vi "Blocking Read After Fulfill.vi"(8 "error in (no error)":errorcluster) -> (0 "error out":errorcluster)   [LabVIEW 2017, in "Unit Tests.lvlib"]
uses:
  Unit Tests.lvlib
  f4ded3e2-5877-4285-a1a8-ead4dd134e79.vi
  4e1b5ce0-e1b8-49ea-b8a3-943737b07833.vi
  Promise Future/Promise/Promise.lvclass
  E:/Promise/Promise Future/Future/Future.lvclass
  Promise Future/Promise/Read Future.vi
  Promise Future/Future/Write Future.vi
  Promise Future/Future/Read Value.vi
  Promise Future/Future/Future.lvclass
  <vilib>/addons/_JKI Toolkits/Caraya/classes/Test/Test.lvclass
  <vilib>/addons/_JKI Toolkits/Caraya/classes/Assert/Assert.lvclass
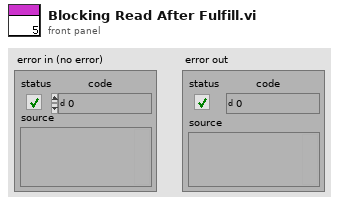
[diagram p1: front panel]
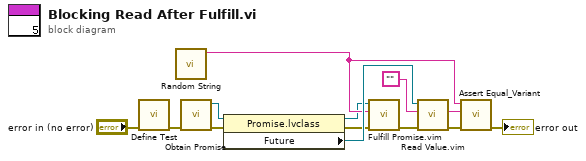
[diagram p0: block diagram]
diagram:
  n1 = call <vilib>:"Define Test.vi"("error in (no error)"="error in (no error)") -> ("error out"=w9:errorcluster)  [unwired: 10 in]
  n2 = call "Random String.vi"() -> ("string"=w7:string)  [unwired: 11 in]
  n3 = call "Obtain Promise.vi"("error in (no error)"=w9) -> ("error out"=w13:errorcluster, "Promise out"=w4:refnum<class "Promise.lvclass">)  [unwired: 8 in, 1 out]
  n4 = property class="Promise.lvclass"(reference=w4, error in=w13) -> (reference out=w3:refnum<class "Promise.lvclass">, error out=w5:errorcluster, "Future"=w12:refnum<class "Future.lvclass">)
  n5 = call "Fulfill Promise.vim"("error in (no error)"=w5, "Value"=w7, "Promise in"=w3) -> ("error out"=w2:errorcluster)  [unwired: 7 in, 1 out]
  n6 = call "Read Value.vim"("error in (no error)"=w2, "Default Value"="", "Future in"=w12) -> ("error out"=w1:errorcluster, "Value"=w6:string)  [unwired: 5 in, 2 out]
  n7 = call <vilib>:"Assert Equal_Variant.vi"("error in (no error)"=w1, "Y"=w6, "X"=w7) -> ("error out"=→"error out":errorcluster)  [unwired: 8 in]
